vi "Meas2 status_1D Arr.vi"(4 "행의 개수":u32, 5 "입력 클러스터":T1, 6 "행 헤더 문자열":string[](array[string])=["S/N"], 8 "에러 입력":errorcluster caption="에러 입력(에러 없음)", 11 "Func_ext":string) -> (0 "에러 출력":errorcluster, 3 "Func_ext Out":string)   [LabVIEW 2020]
uses:
  Controls/Clst_Initialize Input.ctl
  Variables/Global_Cal Info.vi
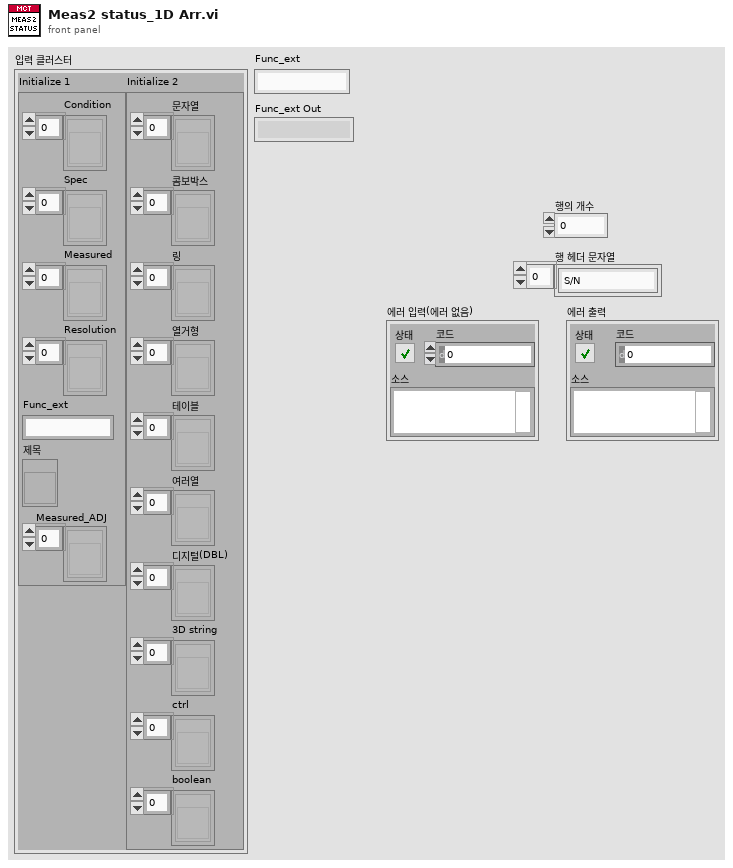
[diagram p1: front panel]
types:
  T1 = typedef "Clst_Initialize Input.ctl" = cluster{"Initialize 1":cluster{"Condition":refnum<vi>[], "Spec":refnum<vi>[], "Measured":refnum<vi>[], "Resolution":refnum<vi>[], "Func_ext":string, "제목":refnum<vi>, "Measured_ADJ":refnum<vi>[]}, "Initialize 2":cluster{"문자열":refnum<vi>[], "콤보박스":refnum<vi>[], "링":refnum<vi>[], "열거형":refnum<vi>[], "테이블":refnum<vi>[], "여러열":refnum<vi>[], "디지털(DBL)":refnum<vi>[], "3D string":refnum<vi>[], "ctrl":refnum<vi>[], "boolean":refnum<vi>[]}}
  T2 = cluster{"세부분류코드":string, "형식":string, "옵션":string, "측정기명":string, "EXCEL파일명":string, "TEMP":string}
  T3 = enum8{"Enabled", "Disabled", "Disabled and Grayed Out"}
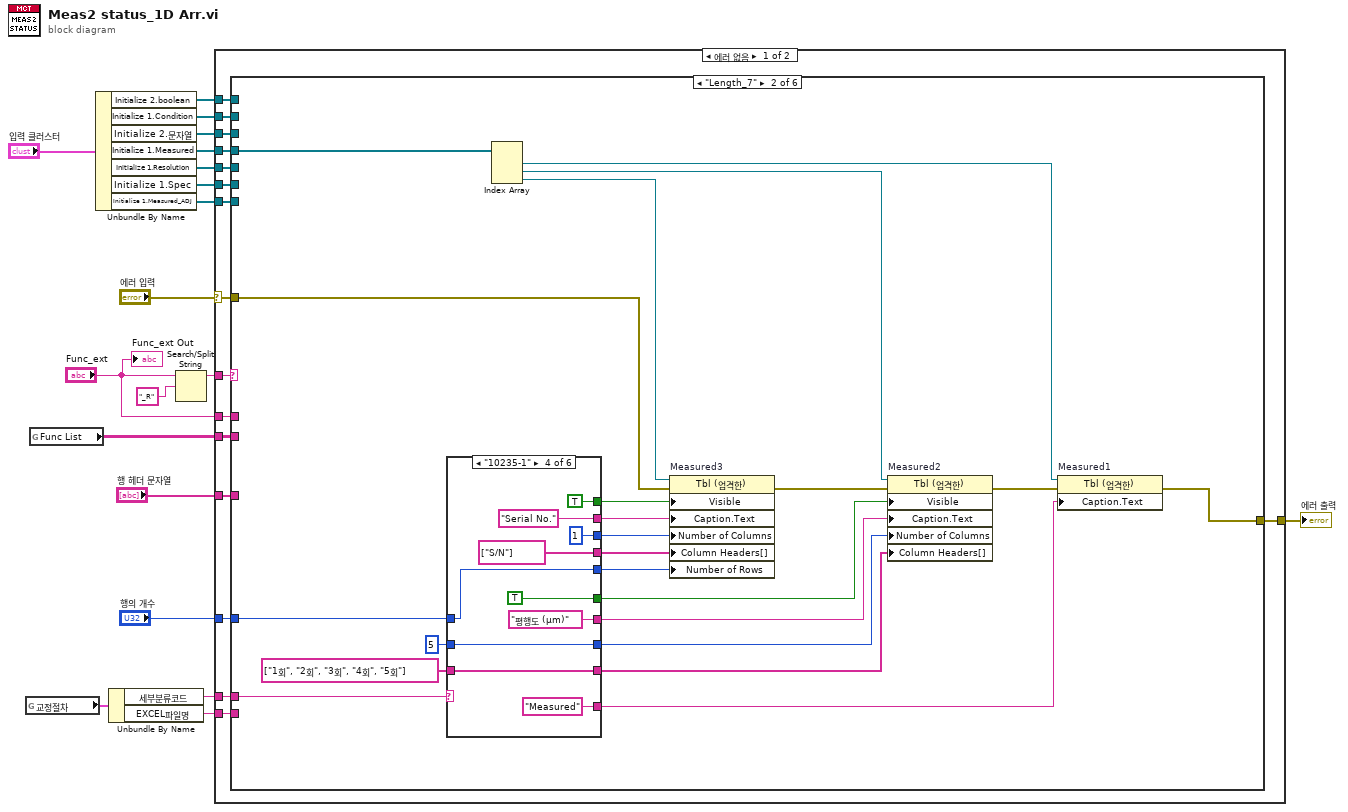
[diagram p0: block diagram]
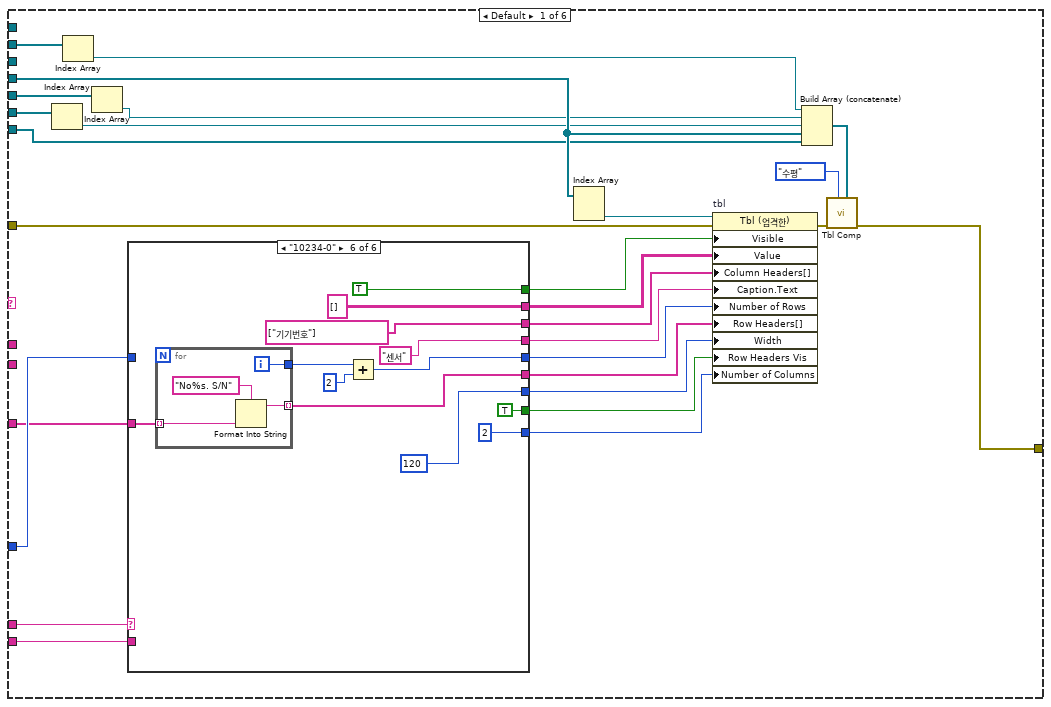
[diagram p2: hidden frame]
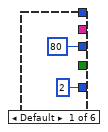
[diagram p3: hidden frame]
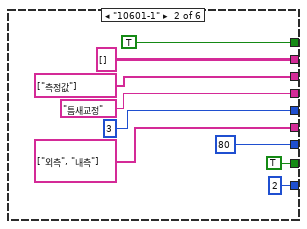
[diagram p4: hidden frame]
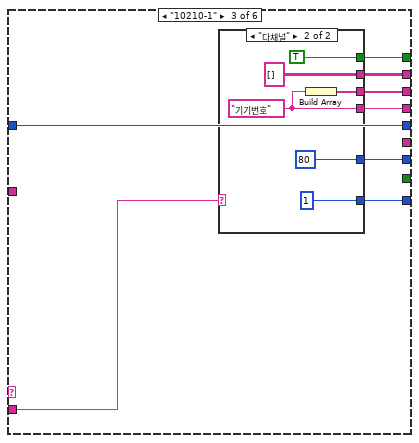
[diagram p5: hidden frame]
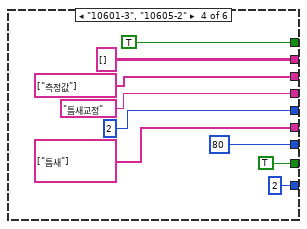
[diagram p7: hidden frame]
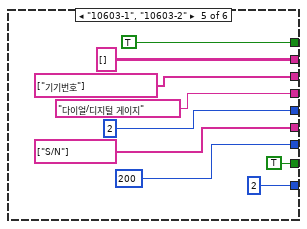
[diagram p8: hidden frame]
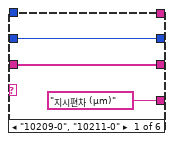
[diagram p9: hidden frame]
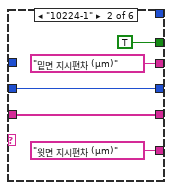
[diagram p10: hidden frame]
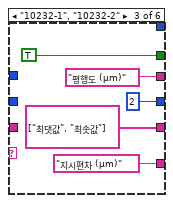
[diagram p11: hidden frame]
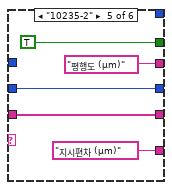
[diagram p12: hidden frame]
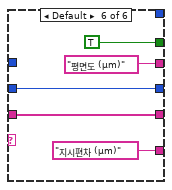
[diagram p13: hidden frame]
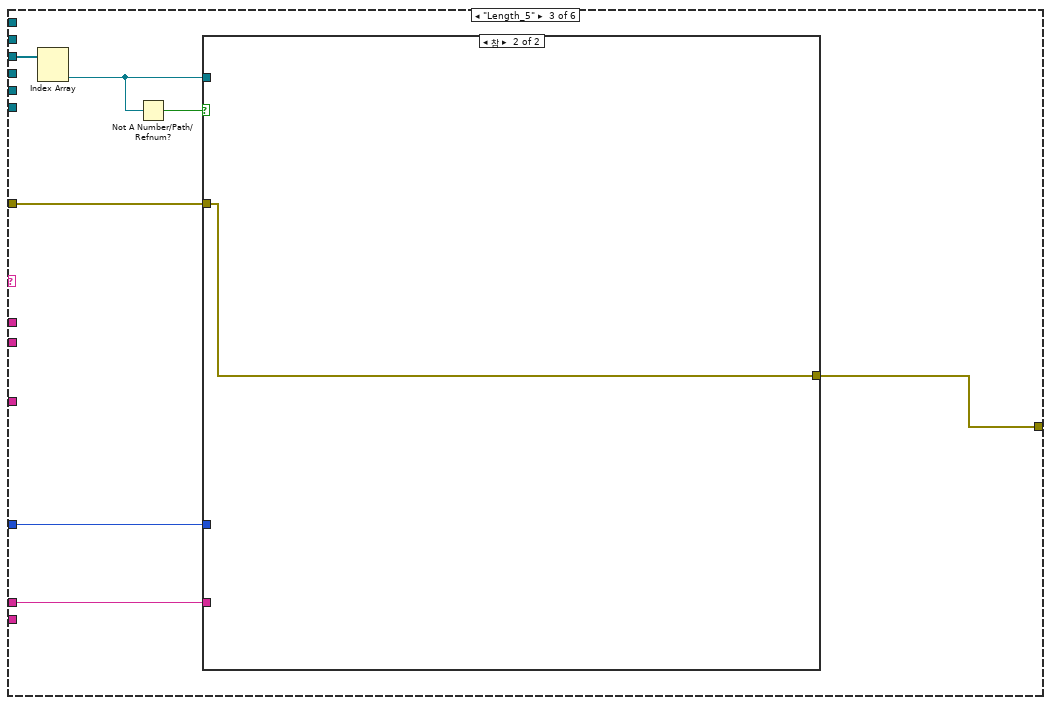
[diagram p14: hidden frame]
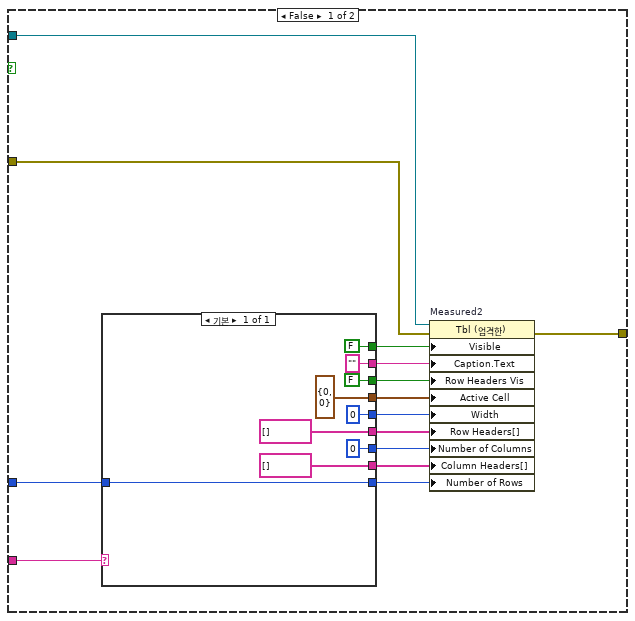
[diagram p15: hidden frame]
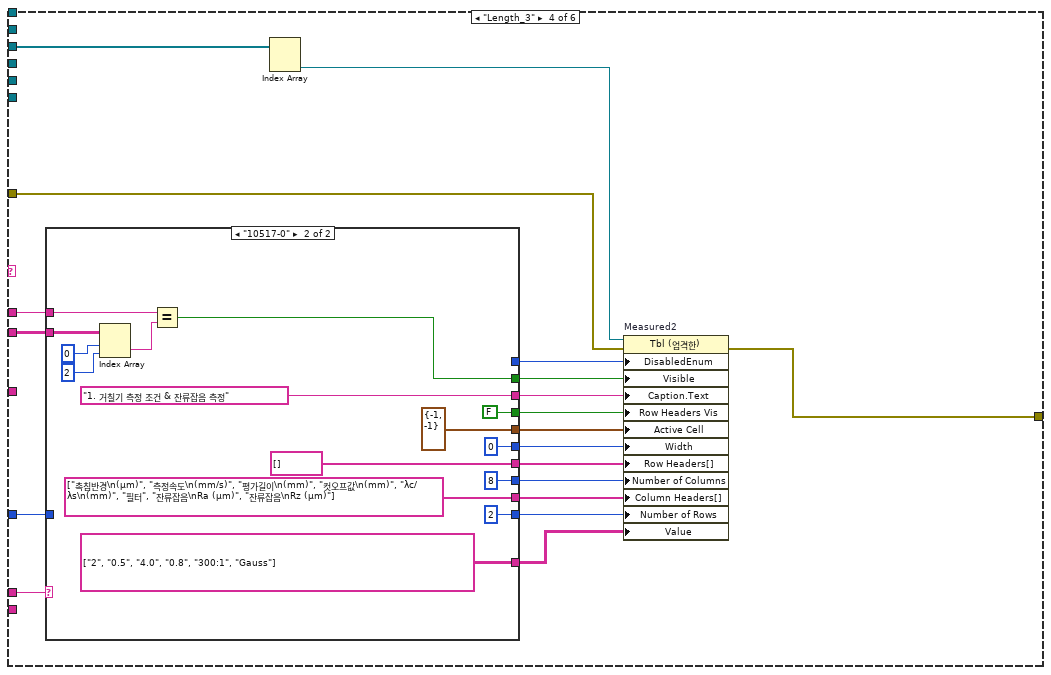
[diagram p16: hidden frame]
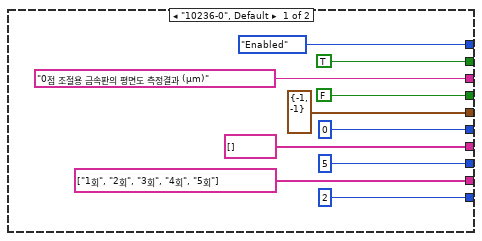
[diagram p17: hidden frame]
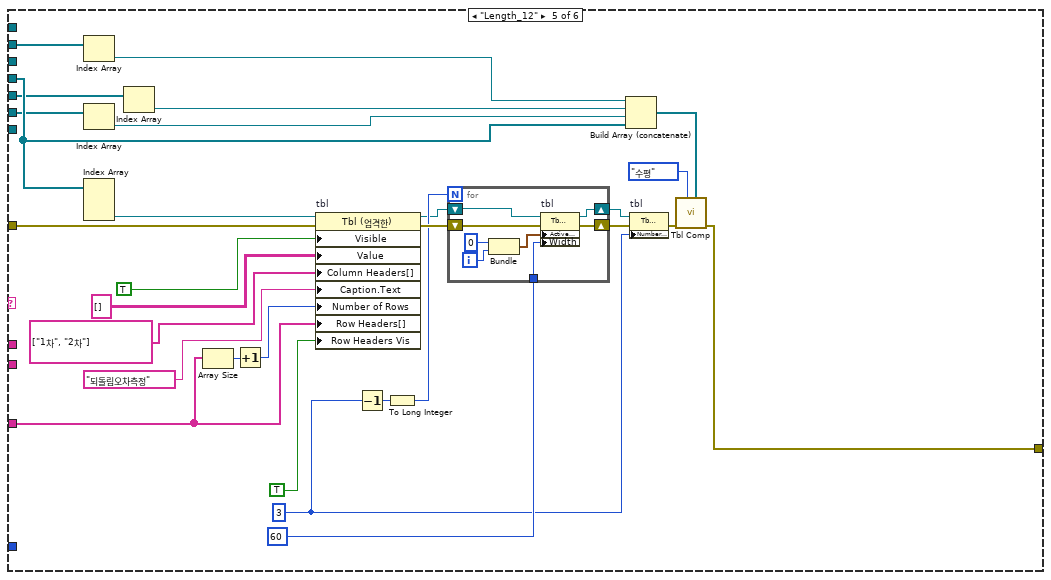
[diagram p18: hidden frame]
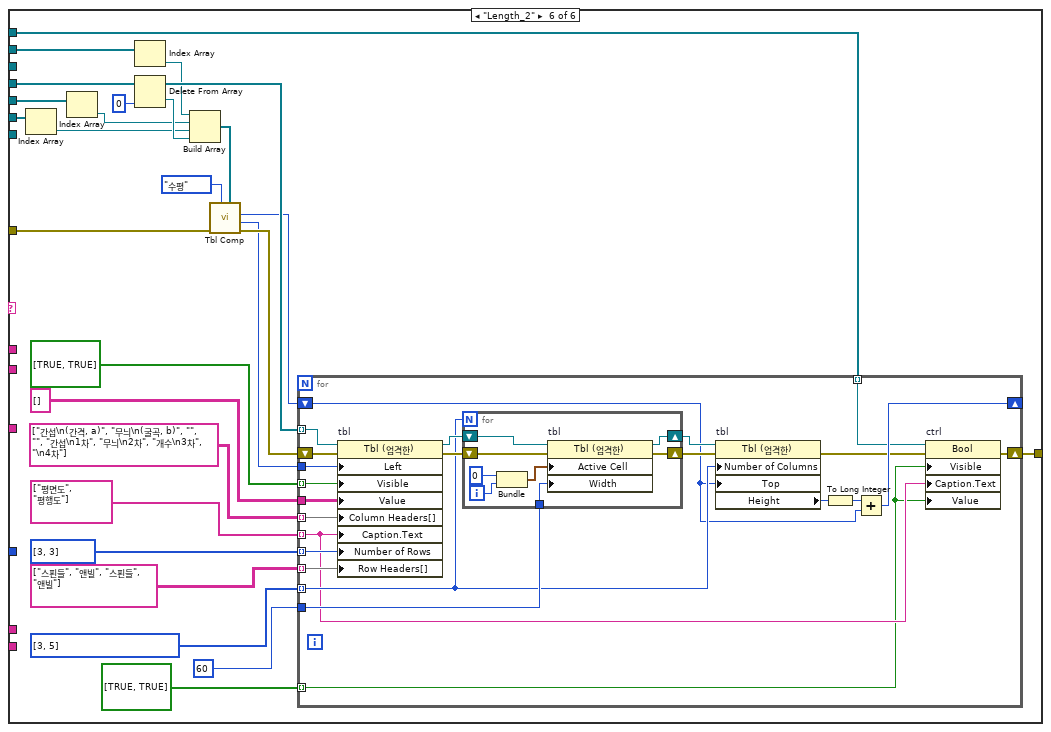
[diagram p19: hidden frame]
diagram:
  n1 = global read "Global_Cal Info.vi" "교정절차"() -> (w17:T2)
  n2 = global read "Global_Cal Info.vi" "Func List"() -> (w2:string[][])
  n3 = Unbundle By Name("입력 클러스터") -> ("Initialize 2.boolean"=w6:refnum<vi>[], "Initialize 1.Condition"=w8:refnum<vi>[], "Initialize 2.문자열"=w5:refnum<vi>[], "Initialize 1.Measured"=w11:refnum<vi>[], "Initialize 1.Resolution"=w10:refnum<vi>[], "Initialize 1.Spec"=w9:refnum<vi>[], "Initialize 1.Measured_ADJ"=w7:refnum<vi>[])
  n4 = Unbundle By Name(w17) -> ("세부분류코드"=w16:string, "EXCEL파일명"=w13:string)
  n5 = Search/Split String(string="Func_ext", search string/char (-)="_R" ("검색 문자열/문자 (-)")) -> (substring before match=w3:string)  [unwired: 1 in, 2 out]
  n6 = case shown="에러 없음" "에러 입력" {
    selector: "에러 입력" -> [w34 w346]
    tunnel: [w35 w346] -> w19
    tunnel: w16 -> [w33 _]
    tunnel: w11 -> [w32 _]
    tunnel: "행의 개수" -> [w31 _]
    tunnel: "행 헤더 문자열" -> [w30 _]
    tunnel: w13 -> [w29 _]
    tunnel: w3 -> [w28 _]
    tunnel: w10 -> [w27 _]
    tunnel: w9 -> [w26 _]
    tunnel: w8 -> [w25 _]
    tunnel: w7 -> [w24 _]
    tunnel: w6 -> [w23 _]
    tunnel: w5 -> [w22 _]
    tunnel: w2 -> [w21 _]
    tunnel: "Func_ext" -> [w20 _]
    frame No Error {
      n7 = case shown="\"Length_7\"" w28 {
        tunnel: [w62 w127 w180 w222 w280 w315] -> w35
        tunnel: w34 -> [w61 w130 w181 w223 w279 w314]
        tunnel: w33 -> [w60 w140 w182 w225 _ _]
        tunnel: w32 -> [w59 w143 w183 w226 w278 w313]
        tunnel: w31 -> [w58 w126 w179 w221 _ _]
        tunnel: w30 -> [w36 _ _ _ w277 _]
        tunnel: w29 -> [w57 _ _ _ _ _]
        tunnel: w27 -> [w41 _ _ _ w256 w296]
        tunnel: w26 -> [w40 _ _ _ w255 w295]
        tunnel: w25 -> [w43 _ _ _ w258 w292]
        tunnel: w24 -> [w56 _ _ _ _ _]
        tunnel: w23 -> [_ _ _ _ _ w289]
        tunnel: w22 -> [_ _ _ _ _ _]
        tunnel: w21 -> [_ _ _ w209 _ _]
        tunnel: w20 -> [_ _ _ w208 _ _]
        frame Default {
          n8 = Index Array(array=w40) -> (element=w38:refnum<vi>)  [unwired: 1 in]
          n9 = Index Array(array=w43) -> (element=w42:refnum<vi>)  [unwired: 1 in]
          n10 = Index Array(array=w41) -> (element=w39:refnum<vi>)  [unwired: 1 in]
          n11 = case shown="\"10234-0\"" w60 {
            tunnel: [_ TRUE ("보이기") w81 TRUE ("보이기") TRUE ("보이기") TRUE ("보이기")] -> w54
            tunnel: [_ string[][] [] ("값") w80 string[][] [] ("값") string[][] [] ("값") string[][] [] ("값")] -> w53
            tunnel: [_ string[] ["측정값"] ("열 헤더 문자열[]") w76 string[] ["측정값"] ("열 헤더 문자열[]") string[] ["기기번호"] ("열 헤더 문자열[]") string[] ["기기번호"] ("열 헤더 문자열[]")] -> w52
            tunnel: [_ "틈새교정" ("캡션.텍스트") w77 "틈새교정" ("캡션.텍스트") "다이얼/디지털 게이지" ("캡션.텍스트") "센서" ("캡션.텍스트")] -> w51
            tunnel: [_ u32 3 ("행의 개수") w75 u32 2 ("행의 개수") u32 2 ("행의 개수") w107] -> w50
            tunnel: [_ string[] ["외측", "내측"] ("열 헤더 문자열[]") _ string[] ["틈새"] ("열 헤더 문자열[]") string[] ["S/N"] ("열 헤더 문자열[]") w109] -> w49
            tunnel: [u32 80 ("활성 셀:셀 크기:폭") u32 80 ("활성 셀:셀 크기:폭") w78 u32 80 ("활성 셀:셀 크기:폭") u32 200 ("활성 셀:셀 크기:폭") u32 120 ("활성 셀:셀 크기:폭")] -> w48
            tunnel: [u32 2 ("열의 개수") u32 2 ("열의 개수") w79 u32 2 ("열의 개수") u32 2 ("열의 개수") u32 2 ("열의 개수")] -> w47
            tunnel: w58 -> [_ _ w75 _ _ _]
            tunnel: [_ TRUE ("보이기") _ TRUE ("보이기") TRUE ("보이기") TRUE ("보이기")] -> w46
            tunnel: w57 -> [_ _ w74 _ _ _]
            tunnel: w36 -> [_ _ _ _ _ w110]
            frame Default {
            }
            frame "10601-1" {
            }
            frame "10210-1" {
              n12 = case shown="\"다채널\"" w74 {
                tunnel: [_ TRUE ("보이기")] -> w81
                tunnel: [_ string[][] [] ("값")] -> w80
                tunnel: [_ u32 1 ("열의 개수")] -> w79
                tunnel: [_ u32 80 ("활성 셀:셀 크기:폭")] -> w78
                tunnel: [_ w83] -> w77
                tunnel: [_ w82] -> w76
                frame Default {
                }
                frame "다채널" {
                  w83 = "기기번호" ("캡션.텍스트")
                  n13 = Build Array(w83) -> (w82:string[])
                }
              }
            }
            frame "10601-3", "10605-2" {
            }
            frame "10603-1", "10603-2" {
            }
            frame "10234-0" {
              n14 = for {
                tunnel: w110 -> [w121] mode=indexing
                tunnel: [w119] -> w109 mode=indexing
                tunnel: [w118] -> w108
                i -> [w118]
                n15 = Format Into String(format string="No%s. S/N", w121) -> (resulting string=w119:string)  [unwired: 2 in, 1 out]
              }
              n16 = Add(x=w108, y=2) -> (x+y=w107:i32)
            }
          }
          n17 = Index Array(array=w59) -> (element #2=w55:refnum<vi>)  [unwired: 2 in, 1 out]
          n18 = property on="tbl" class="Tbl (엄격한)"(reference=w55, error in=w61, "Visible"=w54, "Value"=w53, "Column Headers[]"=w52, "Caption.Text"=w51, "Number of Rows"=w50, "Row Headers[]"=w49, "Width"=w48, "Row Headers Vis"=w46, "Number of Columns"=w47) -> (error out=w45:errorcluster)  [unwired: 1 out]
          n19 = Build Array (concatenate)(w42, w39, w38, w59, w56) -> (w37:refnum<vi>[])
          n20 = call "Tbl Comp.vi"("배열"=w37, "방향"=enum16{"수직", "수평"}."수평", "에러 입력"=w45) -> ("에러 출력"=w62:errorcluster)  [unwired: 6 in, 2 out]
        }
        frame "Length_7" {
          n21 = case shown="\"10235-1\"" w140 {
            tunnel: [_ TRUE TRUE TRUE TRUE TRUE] -> w137
            tunnel: [_ _ _ TRUE _ _] -> w133
            tunnel: [_ "밑면 지시편차 (μm)" "평행도 (μm)" "평행도 (μm)" "평행도 (μm)" "평면도 (μm)"] -> w136
            tunnel: ["지시편차 (μm)" "윗면 지시편차 (μm)" "지시편차 (μm)" "Measured" "지시편차 (μm)" "지시편차 (μm)"] -> w139
            tunnel: [w145 w148 u32 2 w164 w168 w173] -> w135
            tunnel: u32 5 -> [w145 w148 _ w164 w168 w173]
            tunnel: string[] ["1회", "2회", "3회", "4회", "5회"] -> [w144 w147 _ w163 w167 w172]
            tunnel: [w144 w147 string[] ["최댓값", "최솟값"] w163 w167 w172] -> w134
            tunnel: w126 -> [_ _ _ w162 _ _]
            tunnel: [_ _ _ w162 _ _] -> w122
            tunnel: [_ _ _ "Serial No." _ _] -> w125
            tunnel: [_ _ _ u32 1 _ _] -> w124
            tunnel: [_ _ _ string[] ["S/N"] ("열 헤더 문자열[]") _ _] -> w123
            frame "10209-0", "10211-0" {
            }
            frame "10224-1" {
            }
            frame "10232-1", "10232-2" {
            }
            frame "10235-1" {
            }
            frame "10235-2" {
            }
            frame Default {
            }
          }
          n22 = Index Array(array=w143) -> (element #1=w138:refnum<vi>, element #2=w131:refnum<vi>, element #3=w132:refnum<vi>)  [unwired: 3 in]
          n23 = property on="Measured3" class="Tbl (엄격한)"(reference=w132, error in=w130, "Visible"=w133, "Caption.Text"=w125, "Number of Columns"=w124, "Column Headers[]"=w123, "Number of Rows"=w122) -> (error out=w129:errorcluster)  [unwired: 1 out]
          n24 = property on="Measured2" class="Tbl (엄격한)"(reference=w131, error in=w129, "Visible"=w137, "Caption.Text"=w136, "Number of Columns"=w135, "Column Headers[]"=w134) -> (error out=w128:errorcluster)  [unwired: 1 out]
          n25 = property on="Measured1" class="Tbl (엄격한)"(reference=w138, error in=w128, "Caption.Text"=w139) -> (error out=w127:errorcluster)  [unwired: 1 out]
        }
        frame "Length_5" {
          n26 = Index Array(array=w183) -> (element #2=w178:refnum<vi>)  [unwired: 2 in, 1 out]
          n27 = Not A Number/Path/Refnum?(number/path/refnum=w178) -> (NaN/Path/Refnum?=w177:bool)
          n28 = case shown="참" w177 {
            tunnel: w182 -> [w197 _]
            tunnel: w178 -> [w196 _]
            tunnel: w181 -> [w195 w207]
            tunnel: [w194 w207] -> w180
            tunnel: w179 -> [w193 _]
            frame False {
              n29 = case shown="기본" w197 {
                tunnel: w193 -> [w206]
                tunnel: [FALSE] -> w192
                tunnel: [""] -> w191
                tunnel: [w206] -> w189
                tunnel: [string[] [] ("열 헤더 문자열[]")] -> w190
                tunnel: [u32 0] -> w188
                tunnel: [FALSE] -> w187
                tunnel: [cluster{"Row":i32, "Column":i32} {"Row"=0, "Column"=0} ("활성 셀:활성 셀")] -> w186
                tunnel: [u32 0] -> w185
                tunnel: [string[] [] ("행 헤더 문자열[]")] -> w184
                frame 기본 {
                }
              }
              n30 = property on="Measured2" class="Tbl (엄격한)"(reference=w196, error in=w195, "Visible"=w192, "Caption.Text"=w191, "Row Headers Vis"=w187, "Active Cell"=w186, "Width"=w185, "Row Headers[]"=w184, "Number of Columns"=w188, "Column Headers[]"=w190, "Number of Rows"=w189) -> (error out=w194:errorcluster)  [unwired: 1 out]
            }
            frame True {
            }
          }
        }
        frame "Length_3" {
          n31 = case shown="\"10517-0\"" w225 {
            tunnel: w221 -> [_ _]
            tunnel: [TRUE w237] -> w220
            tunnel: ["0점 조절용 금속판의 평면도 측정결과 (μm)" "1. 거칠기 측정 조건 & 잔류잡음 측정"] -> w219
            tunnel: [u32 2 ("행의 개수") u32 2 ("행의 개수")] -> w217
            tunnel: [string[] ["1회", "2회", "3회", "4회", "5회"] ("열 헤더 문자열[]") string[] ["촉침반경\n(μm)", "측정속도\n(mm/s)", "평가길이\n(mm)", "컷오프값\n(mm)", "λc/λs\n(mm)", "필터", "잔류잡음\nRa (μm)", "잔류잡음\nRz (μm)"] ("열 헤더 문자열[]")] -> w218
            tunnel: [u32 5 u32 8] -> w216
            tunnel: [FALSE FALSE] -> w215
            tunnel: [cluster{"Row":i32, "Column":i32} {"Row"=-1, "Column"=-1} ("활성 셀:활성 셀") cluster{"Row":i32, "Column":i32} {"Row"=-1, "Column"=-1} ("활성 셀:활성 셀")] -> w214
            tunnel: [u32 0 u32 0] -> w213
            tunnel: [string[] [] ("행 헤더 문자열[]") string[] [] ("행 헤더 문자열[]")] -> w212
            tunnel: [_ string[][] [["2", "0.5", "4.0", "0.8", "300:1", "Gauss"]] ("값")] -> w211
            tunnel: [T3."Enabled" ("비활성화") _] -> w210
            tunnel: w209 -> [_ w242]
            tunnel: w208 -> [_ w239]
            frame "10236-0", Default {
            }
            frame "10517-0" {
              n32 = Index Array(array=w242, index (row)=0 ("인덱스 (행)"), index (col)=2 ("비활성화된 인덱스 (열)")) -> (element=w238:string)
              n33 = Equal?(x=w239, y=w238) -> (x = y?=w237:bool)
            }
          }
          n34 = Index Array(array=w226) -> (element #2=w224:refnum<vi>)  [unwired: 2 in, 1 out]
          n35 = property on="Measured2" class="Tbl (엄격한)"(reference=w224, error in=w223, "DisabledEnum"=w210, "Visible"=w220, "Caption.Text"=w219, "Row Headers Vis"=w215, "Active Cell"=w214, "Width"=w213, "Row Headers[]"=w212, "Number of Columns"=w216, "Column Headers[]"=w218, "Number of Rows"=w217, "Value"=w211) -> (error out=w222:errorcluster)  [unwired: 1 out]
        }
        frame "Length_12" {
          w262 = u32 3 ("열의 개수")
          n36 = Index Array(array=w258) -> (element=w257:refnum<vi>)  [unwired: 1 in]
          n37 = Index Array(array=w255) -> (element=w253:refnum<vi>)  [unwired: 1 in]
          n38 = Index Array(array=w278) -> (element #3=w276:refnum<vi>)  [unwired: 3 in, 2 out]
          n39 = Index Array(array=w256) -> (element=w254:refnum<vi>)  [unwired: 1 in]
          n40 = Array Size(array=w277) -> (size(s)=w259:i32)
          n41 = Increment(x=w259) -> (x+1=w271:i32)
          n42 = property on="tbl" class="Tbl (엄격한)"(reference=w276, error in=w279, "Visible"=TRUE ("보이기"), "Value"=string[][] [] ("값"), "Column Headers[]"=string[] ["1차", "2차"] ("열 헤더 문자열[]"), "Caption.Text"="되돌림오차측정" ("캡션.텍스트"), "Number of Rows"=w271, "Row Headers[]"=w277, "Row Headers Vis"=TRUE ("보이기")) -> (reference out=w263:refnum<vi>, error out=w269:errorcluster)
          n43 = Decrement(x=w262) -> (x-1=w267:u32)
          n44 = To Long Integer(number=w267) -> (32bit integer=w266:i32)
          n45 = for {
            N: w266 -> [_]
            shift-right: [w287] -> w265
            shift-left: w269 -> [w288]
            tunnel: u32 60 ("활성 셀:셀 크기:폭") -> [w286]
            shift-right: [w282] -> w264
            shift-left: w263 -> [w281]
            i -> [w284]
            n46 = Bundle(0, w284) -> (w285:cluster{i32, i32})  [unwired: 1 in]
            n47 = property on="tbl" class="Tbl (엄격한)"(reference=w281, error in=w288, "Active Cell"=w285, "Width"=w286) -> (reference out=w282:refnum<vi>, error out=w287:errorcluster)
          }
          n48 = Build Array (concatenate)(w257, w254, w253, w278) -> (w252:refnum<vi>[])
          n49 = property on="tbl" class="Tbl (엄격한)"(reference=w264, error in=w265, "Number of Columns"=w262) -> (error out=w260:errorcluster)  [unwired: 1 out]
          n50 = call "Tbl Comp.vi"("배열"=w252, "방향"=enum16{"수직", "수평"}."수평", "에러 입력"=w260) -> ("에러 출력"=w280:errorcluster)  [unwired: 6 in, 2 out]
        }
        frame "Length_2" {
          n51 = Index Array(array=w295) -> (element=w293:refnum<vi>)  [unwired: 1 in]
          n52 = Index Array(array=w296) -> (element=w294:refnum<vi>)  [unwired: 1 in]
          n53 = Index Array(array=w292) -> (element=w291:refnum<vi>)  [unwired: 1 in]
          n54 = Delete From Array(array=w313, index=0 ("인덱스")) -> (deleted portion=w302:refnum<vi>, array with subset deleted=w303:refnum<vi>[])  [unwired: 1 in]
          n55 = Build Array(w291, w294, w293, w302) -> (w290:refnum<vi>[])
          n56 = call "Tbl Comp.vi"("배열"=w290, "방향"=enum16{"수직", "수평"}."수평", "에러 입력"=w314) -> ("에러 출력"=w299:errorcluster, "Right"=w297:i32, "Top"=w298:i32)  [unwired: 6 in]
          n57 = for {
            tunnel: bool[] [TRUE, TRUE] -> [w318] mode=indexing
            tunnel: string[][] [] ("값") -> [w336]
            tunnel: string[][] [["간섭\n(간격, a)", "무늬\n(굴곡, b)", "", ""], ["간섭\n1차", "무늬\n2차", "개수\n3차", "\n4차"]] ("열 헤더 문자열[]") -> [w335] mode=indexing
            tunnel: string[] ["평면도", "평행도"] -> [w317] mode=indexing
            tunnel: u32[] [3, 3] -> [w334] mode=indexing
            tunnel: string[][] [["스핀들", "앤빌"], ["스핀들", "앤빌"]] ("열 헤더 문자열[]") -> [w333] mode=indexing
            tunnel: 60 ("활성 셀:셀 크기:폭") -> [w328]
            tunnel: u32[] [3, 5] -> [w325] mode=indexing
            tunnel: w303 -> [w332] mode=indexing
            shift-right: [w320] -> w315
            shift-left: w299 -> [w337]
            tunnel: w297 -> [w331]
            shift-right: [w321] -> _
            shift-left: w298 -> [w322]
            tunnel: w289 -> [w319] mode=indexing
            tunnel: bool[] [TRUE, TRUE] -> [w316] mode=indexing
            n58 = property on="tbl" class="Tbl (엄격한)"(reference=w332, error in=w337, "Left"=w331, "Visible"=w318, "Value"=w336, "Column Headers[]"=w335, "Caption.Text"=w317, "Number of Rows"=w334, "Row Headers[]"=w333) -> (reference out=w329:refnum<vi>, error out=w330:errorcluster)
            n59 = for {
              N: w325 -> [_]
              shift-right: [w344] -> w327
              shift-left: w330 -> [w345]
              tunnel: w328 -> [w339]
              shift-right: [w338] -> w326
              shift-left: w329 -> [w343]
              i -> [w341]
              n60 = Bundle("활성 셀:셀 크기:폭"=0, w341) -> (w342:cluster{"활성 셀:셀 크기:폭":i32, i32})  [unwired: 1 in]
              n61 = property on="tbl" class="Tbl (엄격한)"(reference=w343, error in=w345, "Active Cell"=w342, "Width"=w339) -> (reference out=w338:refnum<vi>, error out=w344:errorcluster)
            }
            n62 = property on="tbl" class="Tbl (엄격한)"(reference=w326, error in=w327, "Number of Columns"=w325, "Top"=w322) -> (error out=w320:errorcluster, "Height"=w324:u32)  [unwired: 1 out]
            n63 = To Long Integer(number=w324) -> (32bit integer=w323:i32)
            n64 = Add(x=w323, y=w322) -> (x+y=w321:i32)
            n65 = property on="ctrl" class="Bool"(reference=w319, error in=w320, "Visible"=w316, "Caption.Text"=w317, "Value"=w316) -> ()  [unwired: 2 out]
          }
        }
      }
    }
    frame Error {
    }
  }
  "에러 출력" <- w19
  "Func_ext Out" <- "Func_ext"
